vi "Load App.vi"(8 "error in":errorcluster) -> (0 "error out":errorcluster)   [LabVIEW 2015, in "Main.lvlib" / "Main.lvclass"]
uses:
  Main.lvclass
  <vilib>/ActorFramework/Actor/Actor.lvclass
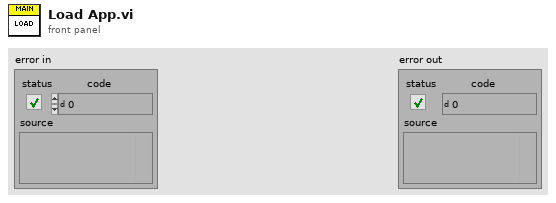
[diagram p1: front panel]
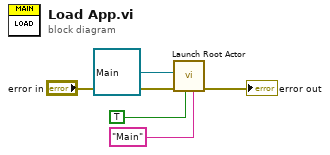
[diagram p0: block diagram]
diagram:
  n1 = call <vilib>:"Launch Root Actor.vi"("Debug Alias"="Main", "Open Actor Core front panel? (F)"=TRUE, "error in"="error in", "Actor"=refnum<class "Main.lvclass"> refnum ("Main.lvlib:Main.lvclass")) -> ("error out"=→"error out":errorcluster)  [unwired: 6 in, 1 out]
